vi "S4GUI_003.vi"(7 "Tab ObsEng":enum32{"Obs", "CCD modes", "Guider", "Eng"}(tab)) -> ()   [LabVIEW 2018] (continued)
            n4857 = call-dynamic "Write Interface.vi"("error in (no error)"=w11578, "Interface.lvclass"=w11579, "Channel in"=w11595) -> ("error out"=w11573:errorcluster, "Channel out"=w11572:refnum<class "Channel.lvclass">)  [unwired: 7 in]
            n4858 = call "Write section_name.vi"("error in (no error)"=w11573, "section_name"="CCD_ACS1", "Channel in"=w11572) -> ("error out"=w11574:errorcluster, "Channel out"=w11569:refnum<class "Channel.lvclass">)  [unwired: 7 in]
            n4859 = call-dynamic "save config.vi"("error in (no error)"=w11574, "file config"="lastsaved.cfg", "Channel in"=w11569) -> ("error out"=w11562:errorcluster, "Channel out"=w11563:refnum<class "Channel.lvclass">)  [unwired: 7 in]
            n4860 = call-dynamic "Read State Machine.vi"("error in (no error)"=w11562, "Device in"=w11563) -> ("error out"=w11577:errorcluster, "State Machine.lvclass"=w11567:refnum<class "State Machine.lvclass">, "Device out"=w11568:refnum<class "Channel.lvclass">)  [unwired: 7 in]
            n4861 = call-dynamic "Write State.vi"("error in (no error)"=w11577, "State"=60, "State Machine in"=w11567) -> ("error out"=w11576:errorcluster, "State Machine out"=w11566:refnum<class "State Machine.lvclass">)  [unwired: 7 in]
            n4862 = call-dynamic "Write State Machine.vi"("error in (no error)"=w11576, "State Machine.lvclass"=w11566, "Device in"=w11568) -> ("error out"=w11564:errorcluster, "Device out"=w11565:refnum<class "Channel.lvclass">)  [unwired: 7 in]
            n4863 = call-dynamic "Write Channel.vi"("error in (no error)"=w11564, "Channel.lvclass"=w11565, "Acquisition in"=w11594) -> ("error out"=w11591:errorcluster, "Acquisition out"=w11590:refnum<class "Acquisition.lvclass">)  [unwired: 7 in]
          }
        }
        n4864 = call-dynamic "Write AcquisitionA.vi"("error in (no error)"=w11298, "Acquisition.lvclass"=w11299, "S4ACS_GUI in"=w11281) -> ("error out"=w11285:errorcluster, "S4ACS_GUI out"=w11280:refnum<class "S4GUI.lvclass">)  [unwired: 7 in]
        n4865 = call "Write AcquisitionB.vi"("error in (no error)"=w11296, "Acquisition.lvclass"=w11297, "S4ACS_GUI in"=w11280) -> ("error out"=w11284:errorcluster, "S4ACS_GUI out"=w11279:refnum<class "S4GUI.lvclass">)  [unwired: 7 in]
        n4866 = call-dynamic "Write AcquisitionC.vi"("error in (no error)"=w11294, "Acquisition.lvclass"=w11295, "S4ACS_GUI in"=w11279) -> ("error out"=w11283:errorcluster, "S4ACS_GUI out"=w11278:refnum<class "S4GUI.lvclass">)  [unwired: 7 in]
        n4867 = call-dynamic "Write AcquisitionD.vi"("error in (no error)"=w11286, "Acquisition.lvclass"=w11287, "S4ACS_GUI in"=w11278) -> ("error out"=w11282:errorcluster, "S4ACS_GUI out"=w11262:refnum<class "S4GUI.lvclass">)  [unwired: 7 in]
        n4868 = Merge Errors(w11285, w11284, w11283, w11282) -> (w11261:errorcluster)
        n4869 = call "Read Instrument.lvclass.vi"("error in (no error)"=w11261, "S4ACS_GUI in"=w11262) -> ("error out"=w11267:errorcluster, "Instrument.lvclass"=w11266:refnum<class "Instrument.lvclass">, "S4ACS_GUI out"=w11263:refnum<class "S4GUI.lvclass">)  [unwired: 7 in]
        n4870 = call "Read ASEL.vi"("error in (no error)"=w11267, "Instrument in"=w11266) -> ("error out"=w11274:errorcluster, "Opt_Selector.lvclass"=w11273:refnum<class "Opt_Selector.lvclass">, "Instrument out"=w11272:refnum<class "Instrument.lvclass">)  [unwired: 7 in]
        n4871 = call "Read target name.vi"("error in (no error)"=w11274, "Optics in"=w11273) -> ("error out"=w11270:errorcluster, "target name"=w11250:string, "Optics out"=w11271:refnum<class "Opt_Selector.lvclass">)  [unwired: 7 in]
        n4872 = call "Write ASEL.vi"("error in (no error)"=w11270, "Opt_Selector.lvclass"=w11271, "Instrument in"=w11272) -> ("error out"=w11269:errorcluster, "Instrument out"=w11265:refnum<class "Instrument.lvclass">)  [unwired: 7 in]
        n4873 = Concatenate Strings(w11252, " ASEL=" ("string"), w11250) -> (w11247:string)
        n4874 = case shown="\"ON\"" w11250 {
          tunnel: w11269 -> [w11416 w11427]
          tunnel: [w11416 w11423] -> w11268
          tunnel: w11265 -> [w11415 w11428]
          tunnel: [w11415 w11424] -> w11264
          frame Default {
          }
          frame "ON" {
            n4875 = call "Read WPROT.vi"("error in (no error)"=w11427, "Instrument in"=w11428) -> ("error out"=w11419:errorcluster, "Opt_Selector.lvclass"=w11426:refnum<class "Opt_Selector.lvclass">, "Instrument out"=w11425:refnum<class "Instrument.lvclass">)  [unwired: 7 in]
            n4876 = call-dynamic "Read sequencia.vi"("error in (no error)"=w11419, "Opt_Selector in"=w11426) -> ("error out"=w11418:errorcluster, "sequencia"=w11422:u16, "Opt_Selector out"=w11421:refnum<class "Opt_Selector.lvclass">)  [unwired: 7 in]
            n4877 = case shown="0" w11422 {
              tunnel: w11421 -> [w11430 w11439]
              tunnel: [w11430 w11435] -> w11420
              tunnel: w11418 -> [w11429 w11438]
              tunnel: [w11429 w11433] -> w11417
              frame Default {
              }
              frame 0 {
                n4878 = call-dynamic "Write sequencia.vi"("error in (no error)"=w11438, "sequencia"=u16 1, "Opt_Selector in"=w11439) -> ("error out"=w11434:errorcluster, "Opt_Selector out"=w11436:refnum<class "Opt_Selector.lvclass">)  [unwired: 7 in]
                n4879 = local write "P0"(TRUE ("P0")) -> ()
                n4880 = call-dynamic "Write sequencia_ant.vi"("error in (no error)"=w11434, "sequencia_ant"=u16 1, "Opt_Selector in"=w11436) -> ("error out"=w11433:errorcluster, "Opt_Selector out"=w11435:refnum<class "Opt_Selector.lvclass">)  [unwired: 7 in]
              }
            }
            n4881 = call "Write WPROT.vi"("error in (no error)"=w11417, "Opt_Selector.lvclass"=w11420, "Instrument in"=w11425) -> ("error out"=w11423:errorcluster, "Instrument out"=w11424:refnum<class "Instrument.lvclass">)  [unwired: 7 in]
          }
        }
        n4882 = call "Write Instrument.lvclass.vi"("error in (no error)"=w11268, "Instrument.lvclass"=w11264, "S4ACS_GUI in"=w11263) -> ("error out"=w11248:errorcluster, "S4ACS_GUI out"=w11249:refnum<class "S4GUI.lvclass">)  [unwired: 7 in]
        n4883 = call-dynamic "Write User Event.vi"("error in (no error)"=w11248, "User Event"=w11247, "S4GUI in"=w11249) -> ("error out"=w11245:errorcluster, "S4GUI out"=w11246:refnum<class "S4GUI.lvclass">)  [unwired: 7 in]
      }
      event "Init mode": Value Change {
        n4884 = event-data() -> ()  [unwired: 1 in, 4 out]
        n4885 = call-dynamic "Write User Event.vi"("error in (no error)"=w11648, "User Event"="INIT INSTRUMENT CLICKED", "S4GUI in"=w11649) -> ("error out"=w11646:errorcluster, "S4GUI out"=w11647:refnum<class "S4GUI.lvclass">)  [unwired: 7 in]
        n4886 = call-dynamic "Read Obs_state.vi"("error in (no error)"=w11646, "S4ACS_GUI in"=w11647) -> ("error out"=w11650:errorcluster, "Obs_state"=w11652:u32, "S4ACS_GUI out"=w11653:refnum<class "S4GUI.lvclass">)  [unwired: 7 in]
        n4887 = In Range and Coerce(upper limit=u32 226, x=w11652, lower limit=u32 220 ("upper limit")) -> (In Range?=w11651:bool)  [unwired: 1 out]
        n4888 = case shown="False" w11651 {
          tunnel: [w11661 w11669] -> w11657
          tunnel: [w11660 w11667] -> w11656
          tunnel: w11650 -> [w11659 w11668]
          tunnel: w11653 -> [w11658 w11670]
          frame False {
            n4889 = call-dynamic "Write sync.vi"("error in (no error)"=w11659, "sync"=TRUE, "S4ACS_GUI in"=w11658) -> ("error out"=w11663:errorcluster, "S4ACS_GUI out"=w11662:refnum<class "S4GUI.lvclass">)  [unwired: 7 in]
            n4890 = call-dynamic "Write Obs_state.vi"("error in (no error)"=w11663, "Obs_state"=u32 220, "S4ACS_GUI in"=w11662) -> ("error out"=w11660:errorcluster, "S4ACS_GUI out"=w11661:refnum<class "S4GUI.lvclass">)  [unwired: 7 in]
          }
          frame True {
            n4891 = call-dynamic "Write Obs_state.vi"("error in (no error)"=w11668, "Obs_state"=u32 0, "S4ACS_GUI in"=w11670) -> ("error out"=w11667:errorcluster, "S4ACS_GUI out"=w11669:refnum<class "S4GUI.lvclass">)  [unwired: 7 in]
          }
        }
      }
      event "exit": Value Change {
        n4892 = event-data() -> ()  [unwired: 1 in, 4 out]
        n4893 = call-dynamic "Read Obs_state.vi"("error in (no error)"=w11674, "S4ACS_GUI in"=w11675) -> ("error out"=w11672:errorcluster, "Obs_state"=w11676:u32, "S4ACS_GUI out"=w11673:refnum<class "S4GUI.lvclass">)  [unwired: 7 in]
        n4894 = In Range and Coerce(upper limit=u32 239, x=w11676, lower limit=u32 230 ("upper limit")) -> (In Range?=w11671:bool)  [unwired: 1 out]
        n4895 = case shown="False" w11671 {
          tunnel: [w11689 w11821] -> w11680
          tunnel: [w11688 w11820] -> w11679
          tunnel: w11673 -> [w11682 w11821]
          tunnel: w11672 -> [w11681 w11820]
          frame False {
            n4896 = call "Read Instrument.lvclass.vi"("error in (no error)"=w11681, "S4ACS_GUI in"=w11682) -> ("error out"=w11683:errorcluster, "Instrument.lvclass"=w11685:refnum<class "Instrument.lvclass">, "S4ACS_GUI out"=w11687:refnum<class "S4GUI.lvclass">)  [unwired: 7 in]
            n4897 = call-dynamic "Read operational.vi"("error in (no error)"=w11683, "Server in"=w11685) -> ("error out"=w11686:errorcluster, "operational"=w11684:bool)  [unwired: 7 in, 1 out]
            n4898 = case shown="True" w11684 {
              tunnel: [w11699 w11767] -> w11689
              tunnel: [w11698 w11766] -> w11688
              tunnel: w11687 -> [w11696 w11765]
              tunnel: w11686 -> [w11697 w11764]
              frame False {
                # "Park condition:\nidle: T\nAND\nall discon: F"
                # "S4ICS not operational: only ACS parking can \nbe allowed, depending on its status..."
                n4899 = call-dynamic "VerifyAcqStatus.vi"("error in (no error)"=w11697, "S4GUI in"=w11696) -> ("error out"=w11691:errorcluster, "idle"=w11695:bool, "S4GUI out"=w11693:refnum<class "S4GUI.lvclass">)  [unwired: 6 in, 1 out]
                n4900 = case shown="True" w11695 {
                  selector: w11695 -> [w11700 _]
                  tunnel: [w11700 w11703] -> w11694
                  tunnel: w11693 -> [w11702 w11707]
                  tunnel: [w11702 w11706] -> w11692
                  tunnel: w11691 -> [w11701 w11705]
                  tunnel: [w11701 w11704] -> w11690
                  frame False {
                  }
                  frame True {
                    n4901 = call-dynamic "VerifAllChanDiscon.vi"("error in (no error)"=w11705, "S4GUI in"=w11707) -> ("error out"=w11704:errorcluster, "All disconnected"=w11708:bool, "S4GUI out"=w11706:refnum<class "S4GUI.lvclass">)  [unwired: 7 in]
                    n4902 = Not(x=w11708) -> (.not. x?=w11703:bool)
                  }
                }
                n4903 = case shown="False" w11694 {
                  tunnel: w11690 -> [w11717 w11736]
                  tunnel: w11692 -> [w11718 w11735]
                  tunnel: [w11711 w11734] -> w11699
                  tunnel: [w11710 w11733] -> w11698
                  frame False {
                    # "Acquisition in progress OR no channel operational..."
                    n4904 = Two Button Dialog(message="Parking not possible.\nAre you sure to quit?", 2:"Yes" ("T button name (\"OK\")")) -> (T button?=w11714:bool)  [unwired: 1 in]
                    n4905 = case shown="True" w11714 {
                      tunnel: [w11721 w11725] -> w11713
                      tunnel: w11718 -> [w11721 w11726]
                      tunnel: w11717 -> [w11720 w11724]
                      tunnel: [w11720 w11723] -> w11712
                      tunnel: ["EXIT CLICKED WITH NO PARKING POSSIBLE. EXIT CANCELLED. " ("T button name (\"OK\")") "EXIT CLICKED WITH NO PARKING POSSIBLE." ("T button name (\"OK\")")] -> w11709
                      frame False {
                        # "NO (cancel)"
                      }
                      frame True {
                        # "YES"
                        n4906 = call-dynamic "Write exit.vi"("error in (no error)"=w11724, "exit"=TRUE, "S4GUI in"=w11726) -> ("error out"=w11723:errorcluster, "S4GUI out"=w11725:refnum<class "S4GUI.lvclass">)  [unwired: 7 in]
                      }
                    }
                    n4907 = call-dynamic "Write User Event.vi"("error in (no error)"=w11712, "User Event"=w11709, "S4GUI in"=w11713) -> ("error out"=w11710:errorcluster, "S4GUI out"=w11711:refnum<class "S4GUI.lvclass">)  [unwired: 7 in]
                  }
                  frame True {
                    # "No acquisition in progress."
                    n4908 = call <vilib>:"Three Button Dialog.vi"("Right Button Text (\"Cancel\")"="Cancel" ("Right Button Text (\"Cancel\")"), "Center Button Text (\"No\")"="NO" ("F button name (\"Cancel\")"), "Left Button Text (\"Yes\")"="YES" ("T button name (\"OK\")"), "message"="Instrument parking not possible.\nPark acquisition system before exiting?") -> ("Which Button?"=w11731:T34)  [unwired: 7 in]
                    n4909 = case shown="\"Right Button\", Default" w11731 {
                      tunnel: w11736 -> [w11743 w11747 w11756]
                      tunnel: w11735 -> [w11742 w11748 w11755]
                      tunnel: [w11739 w11746 w11752] -> w11734
                      tunnel: [w11737 w11745 w11750] -> w11733
                      frame "Center Button" {
                        # "NO"
                        n4910 = call-dynamic "Write exit.vi"("error in (no error)"=w11743, "exit"=TRUE, "S4GUI in"=w11742) -> ("error out"=w11738:errorcluster, "S4GUI out"=w11740:refnum<class "S4GUI.lvclass">)  [unwired: 7 in]
                        n4911 = call-dynamic "Write User Event.vi"("error in (no error)"=w11738, "User Event"="EXIT APP CLICKED WITH NO PARKING.", "S4GUI in"=w11740) -> ("error out"=w11737:errorcluster, "S4GUI out"=w11739:refnum<class "S4GUI.lvclass">)  [unwired: 7 in]
                      }
                      frame "Right Button", Default {
                        # "CANCEL"
                        n4912 = call-dynamic "Write User Event.vi"("error in (no error)"=w11747, "User Event"="EXIT APP CLICKED, BUT CANCELLED BY USER.", "S4GUI in"=w11748) -> ("error out"=w11745:errorcluster, "S4GUI out"=w11746:refnum<class "S4GUI.lvclass">)  [unwired: 7 in]
                      }
                      frame "Left Button" {
                        # "YES"
                        n4913 = call-dynamic "Write sync.vi"("error in (no error)"=w11756, "sync"=TRUE, "S4ACS_GUI in"=w11755) -> ("error out"=w11758:errorcluster, "S4ACS_GUI out"=w11757:refnum<class "S4GUI.lvclass">)  [unwired: 7 in]
                        n4914 = call-dynamic "Write Obs_state.vi"("error in (no error)"=w11758, "Obs_state"=u32 232, "S4ACS_GUI in"=w11757) -> ("error out"=w11751:errorcluster, "S4ACS_GUI out"=w11753:refnum<class "S4GUI.lvclass">)  [unwired: 7 in]
                        n4915 = call-dynamic "Write User Event.vi"("error in (no error)"=w11751, "User Event"="EXIT APP CLICKED AND ONLY ACS PARKING PROCEDURE DONE.", "S4GUI in"=w11753) -> ("error out"=w11750:errorcluster, "S4GUI out"=w11752:refnum<class "S4GUI.lvclass">)  [unwired: 7 in]
                      }
                    }
                  }
                }
              }
              frame True {
                # "Park condition:\nidle: T"
                # "S4ICS operational: Instrument parking allowed \nand verifying ACS channels status..."
                n4916 = call-dynamic "VerifyAcqStatus.vi"("error in (no error)"=w11764, "S4GUI in"=w11765) -> ("error out"=w11761:errorcluster, "idle"=w11762:bool, "S4GUI out"=w11763:refnum<class "S4GUI.lvclass">)  [unwired: 6 in, 1 out]
                n4917 = case shown="False" w11762 {
                  tunnel: [w11771 w11795] -> w11767
                  tunnel: [w11770 w11794] -> w11766
                  tunnel: w11763 -> [w11769 w11788]
                  tunnel: w11761 -> [w11768 w11787]
                  frame False {
                    # "Acquisition in progress..."
                    n4918 = Two Button Dialog(message="Parking not possible.\nAre you sure to quit?", 2:"Yes" ("T button name (\"OK\")")) -> (T button?=w11775:bool)  [unwired: 1 in]
                    n4919 = case shown="True" w11775 {
                      tunnel: [w11780 w11784] -> w11774
                      tunnel: w11769 -> [w11780 w11785]
                      tunnel: w11768 -> [w11779 w11783]
                      tunnel: [w11779 w11782] -> w11773
                      tunnel: ["EXIT CLICKED WITH NO PARKING POSSIBLE. EXIT CANCELLED. " ("T button name (\"OK\")") "EXIT CLICKED WITH NO PARKING POSSIBLE." ("T button name (\"OK\")")] -> w11772
                      frame False {
                        # "NO (cancel)"
                      }
                      frame True {
                        # "YES"
                        n4920 = call-dynamic "Write exit.vi"("error in (no error)"=w11783, "exit"=TRUE, "S4GUI in"=w11785) -> ("error out"=w11782:errorcluster, "S4GUI out"=w11784:refnum<class "S4GUI.lvclass">)  [unwired: 7 in]
                      }
                    }
                    n4921 = call-dynamic "Write User Event.vi"("error in (no error)"=w11773, "User Event"=w11772, "S4GUI in"=w11774) -> ("error out"=w11770:errorcluster, "S4GUI out"=w11771:refnum<class "S4GUI.lvclass">)  [unwired: 7 in]
                  }
                  frame True {
                    # "Acquisition system in IDLE state."
                    n4922 = call <vilib>:"Three Button Dialog.vi"("Right Button Text (\"Cancel\")"="Cancel" ("Right Button Text (\"Cancel\")"), "Center Button Text (\"No\")"="NO" ("F button name (\"Cancel\")"), "Left Button Text (\"Yes\")"="YES" ("T button name (\"OK\")"), "message"="Park before exiting?") -> ("Which Button?"=w11790:T34)  [unwired: 7 in]
                    n4923 = case shown="\"Left Button\"" w11790 {
                      tunnel: w11787 -> [w11802 w11806 w11816]
                      tunnel: w11788 -> [w11801 w11807 w11815]
                      tunnel: [w11798 w11805 w11812] -> w11795
                      tunnel: [w11796 w11804 w11810] -> w11794
                      frame "Center Button" {
                        # "NO"
                        n4924 = call-dynamic "Write exit.vi"("error in (no error)"=w11802, "exit"=TRUE, "S4GUI in"=w11801) -> ("error out"=w11797:errorcluster, "S4GUI out"=w11799:refnum<class "S4GUI.lvclass">)  [unwired: 7 in]
                        n4925 = call-dynamic "Write User Event.vi"("error in (no error)"=w11797, "User Event"="EXIT APP CLICKED WITH NO PARKING.", "S4GUI in"=w11799) -> ("error out"=w11796:errorcluster, "S4GUI out"=w11798:refnum<class "S4GUI.lvclass">)  [unwired: 7 in]
                      }
                      frame "Right Button", Default {
                        # "CANCEL"
                        n4926 = call-dynamic "Write User Event.vi"("error in (no error)"=w11806, "User Event"="EXIT APP CLICKED, BUT CANCELLED BY USER.", "S4GUI in"=w11807) -> ("error out"=w11804:errorcluster, "S4GUI out"=w11805:refnum<class "S4GUI.lvclass">)  [unwired: 7 in]
                      }
                      frame "Left Button" {
                        # "YES"
                        n4927 = call-dynamic "Write sync.vi"("error in (no error)"=w11816, "sync"=TRUE, "S4ACS_GUI in"=w11815) -> ("error out"=w11818:errorcluster, "S4ACS_GUI out"=w11817:refnum<class "S4GUI.lvclass">)  [unwired: 7 in]
                        n4928 = call-dynamic "Write Obs_state.vi"("error in (no error)"=w11818, "Obs_state"=u32 230, "S4ACS_GUI in"=w11817) -> ("error out"=w11811:errorcluster, "S4ACS_GUI out"=w11813:refnum<class "S4GUI.lvclass">)  [unwired: 7 in]
                        n4929 = call-dynamic "Write User Event.vi"("error in (no error)"=w11811, "User Event"="EXIT APP CLICKED AND PARKING PROCEDURE DONE.", "S4GUI in"=w11813) -> ("error out"=w11810:errorcluster, "S4GUI out"=w11812:refnum<class "S4GUI.lvclass">)  [unwired: 7 in]
                      }
                    }
                  }
                }
              }
            }
          }
          frame True {
            # "Parking already in progress..."
          }
        }
      }
      event "WPSEL_stop": Value Change {
        n4930 = event-data() -> ()  [unwired: 1 in, 4 out]
        n4931 = call "Read Instrument.lvclass.vi"("error in (no error)"=w11840, "S4ACS_GUI in"=w11841) -> ("error out"=w11838:errorcluster, "Instrument.lvclass"=w11839:refnum<class "Instrument.lvclass">, "S4ACS_GUI out"=w11825:refnum<class "S4GUI.lvclass">)  [unwired: 7 in]
        n4932 = call "Read WPSEL.vi"("error in (no error)"=w11838, "Instrument in"=w11839) -> ("error out"=w11834:errorcluster, "Opt_Selector.lvclass"=w11837:refnum<class "Opt_Selector.lvclass">, "Instrument out"=w11828:refnum<class "Instrument.lvclass">)  [unwired: 7 in]
        n4933 = call-dynamic "Read State Machine.vi"("error in (no error)"=w11834, "Device in"=w11837) -> ("error out"=w11833:errorcluster, "State Machine.lvclass"=w11836:refnum<class "State Machine.lvclass">, "Device out"=w11830:refnum<class "Opt_Selector.lvclass">)  [unwired: 7 in]
        n4934 = call "Next State.vi"("error in (no error)"=w11833, "New_State"=10, "State Machine in"=w11836) -> ("error out"=w11832:errorcluster, "State Machine out"=w11831:refnum<class "State Machine.lvclass">)  [unwired: 7 in]
        n4935 = call-dynamic "Write State Machine.vi"("error in (no error)"=w11832, "State Machine.lvclass"=w11831, "Device in"=w11830) -> ("error out"=w11827:errorcluster, "Device out"=w11829:refnum<class "Opt_Selector.lvclass">)  [unwired: 7 in]
        n4936 = call "Write WPSEL.vi"("error in (no error)"=w11827, "Opt_Selector.lvclass"=w11829, "Instrument in"=w11828) -> ("error out"=w11824:errorcluster, "Instrument out"=w11826:refnum<class "Instrument.lvclass">)  [unwired: 7 in]
        n4937 = call "Write Instrument.lvclass.vi"("error in (no error)"=w11824, "Instrument.lvclass"=w11826, "S4ACS_GUI in"=w11825) -> ("error out"=w11823:errorcluster, "S4ACS_GUI out"=w11822:refnum<class "S4GUI.lvclass">)  [unwired: 7 in]
      }
      event "WPSEL_init": Value Change {
        n4938 = event-data() -> ()  [unwired: 1 in, 4 out]
        n4939 = call "Read Instrument.lvclass.vi"("error in (no error)"=w11860, "S4ACS_GUI in"=w11861) -> ("error out"=w11858:errorcluster, "Instrument.lvclass"=w11859:refnum<class "Instrument.lvclass">, "S4ACS_GUI out"=w11845:refnum<class "S4GUI.lvclass">)  [unwired: 7 in]
        n4940 = call "Read WPSEL.vi"("error in (no error)"=w11858, "Instrument in"=w11859) -> ("error out"=w11854:errorcluster, "Opt_Selector.lvclass"=w11857:refnum<class "Opt_Selector.lvclass">, "Instrument out"=w11848:refnum<class "Instrument.lvclass">)  [unwired: 7 in]
        n4941 = call-dynamic "Read State Machine.vi"("error in (no error)"=w11854, "Device in"=w11857) -> ("error out"=w11853:errorcluster, "State Machine.lvclass"=w11856:refnum<class "State Machine.lvclass">, "Device out"=w11850:refnum<class "Opt_Selector.lvclass">)  [unwired: 7 in]
        n4942 = call "Next State.vi"("error in (no error)"=w11853, "New_State"=30, "State Machine in"=w11856) -> ("error out"=w11852:errorcluster, "State Machine out"=w11851:refnum<class "State Machine.lvclass">)  [unwired: 7 in]
        n4943 = call-dynamic "Write State Machine.vi"("error in (no error)"=w11852, "State Machine.lvclass"=w11851, "Device in"=w11850) -> ("error out"=w11847:errorcluster, "Device out"=w11849:refnum<class "Opt_Selector.lvclass">)  [unwired: 7 in]
        n4944 = call "Write WPSEL.vi"("error in (no error)"=w11847, "Opt_Selector.lvclass"=w11849, "Instrument in"=w11848) -> ("error out"=w11844:errorcluster, "Instrument out"=w11846:refnum<class "Instrument.lvclass">)  [unwired: 7 in]
        n4945 = call "Write Instrument.lvclass.vi"("error in (no error)"=w11844, "Instrument.lvclass"=w11846, "S4ACS_GUI in"=w11845) -> ("error out"=w11843:errorcluster, "S4ACS_GUI out"=w11842:refnum<class "S4GUI.lvclass">)  [unwired: 7 in]
      }
      event "GMIR_target": Value Change {
        n4946 = event-data() -> ("NewVal"=w11871:dbl)  [unwired: 1 in, 3 out]
        n4947 = call "Read Instrument.lvclass.vi"("error in (no error)"=w11875, "S4ACS_GUI in"=w11876) -> ("error out"=w11873:errorcluster, "Instrument.lvclass"=w11874:refnum<class "Instrument.lvclass">, "S4ACS_GUI out"=w11865:refnum<class "S4GUI.lvclass">)  [unwired: 7 in]
        n4948 = call "Read GMIR.vi"("error in (no error)"=w11873, "Instrument in"=w11874) -> ("error out"=w11870:errorcluster, "Opt_Continuous.lvclass"=w11872:refnum<class "Opt_Continuous.lvclass">, "Instrument out"=w11868:refnum<class "Instrument.lvclass">)  [unwired: 7 in]
        n4949 = call "Write target.vi"("error in (no error)"=w11870, "target"=w11871, "Optics in"=w11872) -> ("error out"=w11867:errorcluster, "Optics out"=w11869:refnum<class "Opt_Continuous.lvclass">)  [unwired: 7 in]
        n4950 = call "Write GMIR.vi"("error in (no error)"=w11867, "Opt_Continuous.lvclass"=w11869, "Instrument in"=w11868) -> ("error out"=w11864:errorcluster, "Instrument out"=w11866:refnum<class "Instrument.lvclass">)  [unwired: 7 in]
        n4951 = call "Write Instrument.lvclass.vi"("error in (no error)"=w11864, "Instrument.lvclass"=w11866, "S4ACS_GUI in"=w11865) -> ("error out"=w11863:errorcluster, "S4ACS_GUI out"=w11862:refnum<class "S4GUI.lvclass">)  [unwired: 7 in]
      }
      event "GMIR_target 2": Value Change {
        n4952 = event-data() -> ("NewVal"=w11878:dbl)  [unwired: 1 in, 3 out]
        n4953 = call-dynamic "Read GSserver.lvclass.vi"("error in (no error)"=w11891, "S4GUI in"=w11892) -> ("error out"=w11889:errorcluster, "GSserver.lvclass"=w11890:refnum<class "GSserver.lvclass">, "S4GUI out"=w11886:refnum<class "S4GUI.lvclass">)  [unwired: 7 in]
        n4954 = call-dynamic "Read Mirror.vi"("error in (no error)"=w11889, "GSserver in"=w11890) -> ("error out"=w11880:errorcluster, "GSdevice.lvclass"=w11882:refnum<class "GSdevice.lvclass">, "GSserver out"=w11888:refnum<class "GSserver.lvclass">)  [unwired: 7 in]
        n4955 = Number To Fractional String(number=w11878) -> (F-format string=w11877:string)  [unwired: 3 in]
        n4956 = call-dynamic "Write target.vi"("error in (no error)"=w11880, "target"=w11877, "GSdevice in"=w11882) -> ("error out"=w11879:errorcluster, "GSdevice out"=w11881:refnum<class "GSdevice.lvclass">)  [unwired: 7 in]
        n4957 = call-dynamic "Write Mirror.vi"("error in (no error)"=w11879, "GSdevice.lvclass"=w11881, "GSserver in"=w11888) -> ("error out"=w11885:errorcluster, "GSserver out"=w11887:refnum<class "GSserver.lvclass">)  [unwired: 7 in]
        n4958 = call-dynamic "Write GSserver.lvclass.vi"("error in (no error)"=w11885, "GSserver.lvclass"=w11887, "S4GUI in"=w11886) -> ("error out"=w11884:errorcluster, "S4GUI out"=w11883:refnum<class "S4GUI.lvclass">)  [unwired: 7 in]
      }
      event "GMIR_set": Value Change {
        n4959 = event-data() -> ()  [unwired: 1 in, 4 out]
        n4960 = call "Read Instrument.lvclass.vi"("error in (no error)"=w11911, "S4ACS_GUI in"=w11912) -> ("error out"=w11909:errorcluster, "Instrument.lvclass"=w11910:refnum<class "Instrument.lvclass">, "S4ACS_GUI out"=w11898:refnum<class "S4GUI.lvclass">)  [unwired: 7 in]
        n4961 = call "Read GMIR.vi"("error in (no error)"=w11909, "Instrument in"=w11910) -> ("error out"=w11906:errorcluster, "Opt_Continuous.lvclass"=w11908:refnum<class "Opt_Continuous.lvclass">, "Instrument out"=w11900:refnum<class "Instrument.lvclass">)  [unwired: 7 in]
        n4962 = call-dynamic "Read State Machine.vi"("error in (no error)"=w11906, "Device in"=w11908) -> ("error out"=w11905:errorcluster, "State Machine.lvclass"=w11896:refnum<class "State Machine.lvclass">, "Device out"=w11902:refnum<class "Opt_Continuous.lvclass">)  [unwired: 7 in]
        n4963 = call "Next State.vi"("error in (no error)"=w11905, "New_State"=1, "State Machine in"=w11896) -> ("error out"=w11904:errorcluster, "State Machine out"=w11903:refnum<class "State Machine.lvclass">)  [unwired: 7 in]
        n4964 = call-dynamic "Write State Machine.vi"("error in (no error)"=w11904, "State Machine.lvclass"=w11903, "Device in"=w11902) -> ("error out"=w11899:errorcluster, "Device out"=w11901:refnum<class "Opt_Continuous.lvclass">)  [unwired: 7 in]
        n4965 = call "Write GMIR.vi"("error in (no error)"=w11899, "Opt_Continuous.lvclass"=w11901, "Instrument in"=w11900) -> ("error out"=w11893:errorcluster, "Instrument out"=w11894:refnum<class "Instrument.lvclass">)  [unwired: 7 in]
        n4966 = call "Write Instrument.lvclass.vi"("error in (no error)"=w11893, "Instrument.lvclass"=w11894, "S4ACS_GUI in"=w11898) -> ("error out"=w11897:errorcluster, "S4ACS_GUI out"=w11895:refnum<class "S4GUI.lvclass">)  [unwired: 7 in]
      }
      event "GMIR_set 2": Value Change {
        n4967 = event-data() -> ()  [unwired: 1 in, 4 out]
        n4968 = call-dynamic "Read GSserver.lvclass.vi"("error in (no error)"=w11931, "S4GUI in"=w11932) -> ("error out"=w11929:errorcluster, "GSserver.lvclass"=w11930:refnum<class "GSserver.lvclass">, "S4GUI out"=w11918:refnum<class "S4GUI.lvclass">)  [unwired: 7 in]
        n4969 = call-dynamic "Read Mirror.vi"("error in (no error)"=w11929, "GSserver in"=w11930) -> ("error out"=w11926:errorcluster, "GSdevice.lvclass"=w11928:refnum<class "GSdevice.lvclass">, "GSserver out"=w11920:refnum<class "GSserver.lvclass">)  [unwired: 7 in]
        n4970 = call-dynamic "Read State Machine.vi"("error in (no error)"=w11926, "Device in"=w11928) -> ("error out"=w11925:errorcluster, "State Machine.lvclass"=w11916:refnum<class "State Machine.lvclass">, "Device out"=w11922:refnum<class "GSdevice.lvclass">)  [unwired: 7 in]
        n4971 = call "Next State.vi"("error in (no error)"=w11925, "New_State"=10, "State Machine in"=w11916) -> ("error out"=w11924:errorcluster, "State Machine out"=w11923:refnum<class "State Machine.lvclass">)  [unwired: 7 in]
        n4972 = call-dynamic "Write State Machine.vi"("error in (no error)"=w11924, "State Machine.lvclass"=w11923, "Device in"=w11922) -> ("error out"=w11919:errorcluster, "Device out"=w11921:refnum<class "GSdevice.lvclass">)  [unwired: 7 in]
        n4973 = call-dynamic "Write Mirror.vi"("error in (no error)"=w11919, "GSdevice.lvclass"=w11921, "GSserver in"=w11920) -> ("error out"=w11913:errorcluster, "GSserver out"=w11914:refnum<class "GSserver.lvclass">)  [unwired: 7 in]
        n4974 = call-dynamic "Write GSserver.lvclass.vi"("error in (no error)"=w11913, "GSserver.lvclass"=w11914, "S4GUI in"=w11918) -> ("error out"=w11917:errorcluster, "S4GUI out"=w11915:refnum<class "S4GUI.lvclass">)  [unwired: 7 in]
      }
      event "GMIR_stop", "GMIR_stop 2": Value Change {
        n4975 = event-data() -> ()  [unwired: 1 in, 4 out]
        n4976 = call "Read Instrument.lvclass.vi"("error in (no error)"=w11951, "S4ACS_GUI in"=w11952) -> ("error out"=w11949:errorcluster, "Instrument.lvclass"=w11950:refnum<class "Instrument.lvclass">, "S4ACS_GUI out"=w11936:refnum<class "S4GUI.lvclass">)  [unwired: 7 in]
        n4977 = call "Read GMIR.vi"("error in (no error)"=w11949, "Instrument in"=w11950) -> ("error out"=w11945:errorcluster, "Opt_Continuous.lvclass"=w11948:refnum<class "Opt_Continuous.lvclass">, "Instrument out"=w11939:refnum<class "Instrument.lvclass">)  [unwired: 7 in]
        n4978 = call-dynamic "Read State Machine.vi"("error in (no error)"=w11945, "Device in"=w11948) -> ("error out"=w11944:errorcluster, "State Machine.lvclass"=w11947:refnum<class "State Machine.lvclass">, "Device out"=w11941:refnum<class "Opt_Continuous.lvclass">)  [unwired: 7 in]
        n4979 = call "Next State.vi"("error in (no error)"=w11944, "New_State"=10, "State Machine in"=w11947) -> ("error out"=w11943:errorcluster, "State Machine out"=w11942:refnum<class "State Machine.lvclass">)  [unwired: 7 in]
        n4980 = call-dynamic "Write State Machine.vi"("error in (no error)"=w11943, "State Machine.lvclass"=w11942, "Device in"=w11941) -> ("error out"=w11938:errorcluster, "Device out"=w11940:refnum<class "Opt_Continuous.lvclass">)  [unwired: 7 in]
        n4981 = call "Write GMIR.vi"("error in (no error)"=w11938, "Opt_Continuous.lvclass"=w11940, "Instrument in"=w11939) -> ("error out"=w11935:errorcluster, "Instrument out"=w11937:refnum<class "Instrument.lvclass">)  [unwired: 7 in]
        n4982 = call "Write Instrument.lvclass.vi"("error in (no error)"=w11935, "Instrument.lvclass"=w11937, "S4ACS_GUI in"=w11936) -> ("error out"=w11934:errorcluster, "S4ACS_GUI out"=w11933:refnum<class "S4GUI.lvclass">)  [unwired: 7 in]
      }
      event "GMIR_init": Value Change {
        n4983 = event-data() -> ()  [unwired: 1 in, 4 out]
        n4984 = call "Read Instrument.lvclass.vi"("error in (no error)"=w11971, "S4ACS_GUI in"=w11972) -> ("error out"=w11969:errorcluster, "Instrument.lvclass"=w11970:refnum<class "Instrument.lvclass">, "S4ACS_GUI out"=w11956:refnum<class "S4GUI.lvclass">)  [unwired: 7 in]
        n4985 = call "Read GMIR.vi"("error in (no error)"=w11969, "Instrument in"=w11970) -> ("error out"=w11965:errorcluster, "Opt_Continuous.lvclass"=w11968:refnum<class "Opt_Continuous.lvclass">, "Instrument out"=w11959:refnum<class "Instrument.lvclass">)  [unwired: 7 in]
        n4986 = call-dynamic "Read State Machine.vi"("error in (no error)"=w11965, "Device in"=w11968) -> ("error out"=w11964:errorcluster, "State Machine.lvclass"=w11967:refnum<class "State Machine.lvclass">, "Device out"=w11961:refnum<class "Opt_Continuous.lvclass">)  [unwired: 7 in]
        n4987 = call "Next State.vi"("error in (no error)"=w11964, "New_State"=30, "State Machine in"=w11967) -> ("error out"=w11963:errorcluster, "State Machine out"=w11962:refnum<class "State Machine.lvclass">)  [unwired: 7 in]
        n4988 = call-dynamic "Write State Machine.vi"("error in (no error)"=w11963, "State Machine.lvclass"=w11962, "Device in"=w11961) -> ("error out"=w11958:errorcluster, "Device out"=w11960:refnum<class "Opt_Continuous.lvclass">)  [unwired: 7 in]
        n4989 = call "Write GMIR.vi"("error in (no error)"=w11958, "Opt_Continuous.lvclass"=w11960, "Instrument in"=w11959) -> ("error out"=w11955:errorcluster, "Instrument out"=w11957:refnum<class "Instrument.lvclass">)  [unwired: 7 in]
        n4990 = call "Write Instrument.lvclass.vi"("error in (no error)"=w11955, "Instrument.lvclass"=w11957, "S4ACS_GUI in"=w11956) -> ("error out"=w11954:errorcluster, "S4ACS_GUI out"=w11953:refnum<class "S4GUI.lvclass">)  [unwired: 7 in]
      }
      event "GFOC_target": Value Change {
        n4991 = event-data() -> ("NewVal"=w11982:dbl)  [unwired: 1 in, 3 out]
        n4992 = call "Read Instrument.lvclass.vi"("error in (no error)"=w11986, "S4ACS_GUI in"=w11987) -> ("error out"=w11984:errorcluster, "Instrument.lvclass"=w11985:refnum<class "Instrument.lvclass">, "S4ACS_GUI out"=w11976:refnum<class "S4GUI.lvclass">)  [unwired: 7 in]
        n4993 = call "Read GFOC.vi"("error in (no error)"=w11984, "Instrument in"=w11985) -> ("error out"=w11981:errorcluster, "Opt_Continuous.lvclass"=w11983:refnum<class "Opt_Continuous.lvclass">, "Instrument out"=w11979:refnum<class "Instrument.lvclass">)  [unwired: 7 in]
        n4994 = call "Write target.vi"("error in (no error)"=w11981, "target"=w11982, "Optics in"=w11983) -> ("error out"=w11978:errorcluster, "Optics out"=w11980:refnum<class "Opt_Continuous.lvclass">)  [unwired: 7 in]
        n4995 = call "Write GFOC.vi"("error in (no error)"=w11978, "Opt_Continuous.lvclass"=w11980, "Instrument in"=w11979) -> ("error out"=w11975:errorcluster, "Instrument out"=w11977:refnum<class "Instrument.lvclass">)  [unwired: 7 in]
        n4996 = call "Write Instrument.lvclass.vi"("error in (no error)"=w11975, "Instrument.lvclass"=w11977, "S4ACS_GUI in"=w11976) -> ("error out"=w11974:errorcluster, "S4ACS_GUI out"=w11973:refnum<class "S4GUI.lvclass">)  [unwired: 7 in]
      }
      event "GFOC_target 2": Value Change {
        n4997 = event-data() -> ("NewVal"=w11989:dbl)  [unwired: 1 in, 3 out]
        n4998 = call-dynamic "Read GSserver.lvclass.vi"("error in (no error)"=w12002, "S4GUI in"=w12003) -> ("error out"=w12000:errorcluster, "GSserver.lvclass"=w12001:refnum<class "GSserver.lvclass">, "S4GUI out"=w11993:refnum<class "S4GUI.lvclass">)  [unwired: 7 in]
        n4999 = call-dynamic "Read Focus.vi"("error in (no error)"=w12000, "GSserver in"=w12001) -> ("error out"=w11998:errorcluster, "GSdevice.lvclass"=w11999:refnum<class "GSdevice.lvclass">, "GSserver out"=w11996:refnum<class "GSserver.lvclass">)  [unwired: 7 in]
        n5000 = Number To Fractional String(number=w11989) -> (F-format string=w11988:string)  [unwired: 3 in]
        n5001 = call-dynamic "Write target.vi"("error in (no error)"=w11998, "target"=w11988, "GSdevice in"=w11999) -> ("error out"=w11995:errorcluster, "GSdevice out"=w11997:refnum<class "GSdevice.lvclass">)  [unwired: 7 in]
        n5002 = call-dynamic "Write Focus.vi"("error in (no error)"=w11995, "GSdevice.lvclass"=w11997, "GSserver in"=w11996) -> ("error out"=w11992:errorcluster, "GSserver out"=w11994:refnum<class "GSserver.lvclass">)  [unwired: 7 in]
        n5003 = call-dynamic "Write GSserver.lvclass.vi"("error in (no error)"=w11992, "GSserver.lvclass"=w11994, "S4GUI in"=w11993) -> ("error out"=w11991:errorcluster, "S4GUI out"=w11990:refnum<class "S4GUI.lvclass">)  [unwired: 7 in]
      }
      event "GFOC_set": Value Change {
        n5004 = event-data() -> ()  [unwired: 1 in, 4 out]
        n5005 = call "Read Instrument.lvclass.vi"("error in (no error)"=w12022, "S4ACS_GUI in"=w12023) -> ("error out"=w12020:errorcluster, "Instrument.lvclass"=w12021:refnum<class "Instrument.lvclass">, "S4ACS_GUI out"=w12008:refnum<class "S4GUI.lvclass">)  [unwired: 7 in]
        n5006 = call "Read GFOC.vi"("error in (no error)"=w12020, "Instrument in"=w12021) -> ("error out"=w12017:errorcluster, "Opt_Continuous.lvclass"=w12019:refnum<class "Opt_Continuous.lvclass">, "Instrument out"=w12011:refnum<class "Instrument.lvclass">)  [unwired: 7 in]
        n5007 = call-dynamic "Read State Machine.vi"("error in (no error)"=w12017, "Device in"=w12019) -> ("error out"=w12016:errorcluster, "State Machine.lvclass"=w12005:refnum<class "State Machine.lvclass">, "Device out"=w12013:refnum<class "Opt_Continuous.lvclass">)  [unwired: 7 in]
        n5008 = call "Next State.vi"("error in (no error)"=w12016, "New_State"=1, "State Machine in"=w12005) -> ("error out"=w12015:errorcluster, "State Machine out"=w12014:refnum<class "State Machine.lvclass">)  [unwired: 7 in]
        n5009 = call-dynamic "Write State Machine.vi"("error in (no error)"=w12015, "State Machine.lvclass"=w12014, "Device in"=w12013) -> ("error out"=w12010:errorcluster, "Device out"=w12012:refnum<class "Opt_Continuous.lvclass">)  [unwired: 7 in]
        n5010 = call "Write GFOC.vi"("error in (no error)"=w12010, "Opt_Continuous.lvclass"=w12012, "Instrument in"=w12011) -> ("error out"=w12007:errorcluster, "Instrument out"=w12009:refnum<class "Instrument.lvclass">)  [unwired: 7 in]
        n5011 = call "Write Instrument.lvclass.vi"("error in (no error)"=w12007, "Instrument.lvclass"=w12009, "S4ACS_GUI in"=w12008) -> ("error out"=w12006:errorcluster, "S4ACS_GUI out"=w12004:refnum<class "S4GUI.lvclass">)  [unwired: 7 in]
      }
      event "GFOC_set 2": Value Change {
        n5012 = event-data() -> ()  [unwired: 1 in, 4 out]
        n5013 = call-dynamic "Read GSserver.lvclass.vi"("error in (no error)"=w12042, "S4GUI in"=w12043) -> ("error out"=w12040:errorcluster, "GSserver.lvclass"=w12041:refnum<class "GSserver.lvclass">, "S4GUI out"=w12028:refnum<class "S4GUI.lvclass">)  [unwired: 7 in]
        n5014 = call-dynamic "Read Focus.vi"("error in (no error)"=w12040, "GSserver in"=w12041) -> ("error out"=w12037:errorcluster, "GSdevice.lvclass"=w12039:refnum<class "GSdevice.lvclass">, "GSserver out"=w12031:refnum<class "GSserver.lvclass">)  [unwired: 7 in]
        n5015 = call-dynamic "Read State Machine.vi"("error in (no error)"=w12037, "Device in"=w12039) -> ("error out"=w12036:errorcluster, "State Machine.lvclass"=w12025:refnum<class "State Machine.lvclass">, "Device out"=w12033:refnum<class "GSdevice.lvclass">)  [unwired: 7 in]
        n5016 = call "Next State.vi"("error in (no error)"=w12036, "New_State"=10, "State Machine in"=w12025) -> ("error out"=w12035:errorcluster, "State Machine out"=w12034:refnum<class "State Machine.lvclass">)  [unwired: 7 in]
        n5017 = call-dynamic "Write State Machine.vi"("error in (no error)"=w12035, "State Machine.lvclass"=w12034, "Device in"=w12033) -> ("error out"=w12030:errorcluster, "Device out"=w12032:refnum<class "GSdevice.lvclass">)  [unwired: 7 in]
        n5018 = call-dynamic "Write Focus.vi"("error in (no error)"=w12030, "GSdevice.lvclass"=w12032, "GSserver in"=w12031) -> ("error out"=w12027:errorcluster, "GSserver out"=w12029:refnum<class "GSserver.lvclass">)  [unwired: 7 in]
        n5019 = call-dynamic "Write GSserver.lvclass.vi"("error in (no error)"=w12027, "GSserver.lvclass"=w12029, "S4GUI in"=w12028) -> ("error out"=w12026:errorcluster, "S4GUI out"=w12024:refnum<class "S4GUI.lvclass">)  [unwired: 7 in]
      }
      event "GFOC_stop", "GFOC_stop 2": Value Change {
        n5020 = event-data() -> ()  [unwired: 1 in, 4 out]
        n5021 = call "Read Instrument.lvclass.vi"("error in (no error)"=w12062, "S4ACS_GUI in"=w12063) -> ("error out"=w12060:errorcluster, "Instrument.lvclass"=w12061:refnum<class "Instrument.lvclass">, "S4ACS_GUI out"=w12047:refnum<class "S4GUI.lvclass">)  [unwired: 7 in]
        n5022 = call "Read GFOC.vi"("error in (no error)"=w12060, "Instrument in"=w12061) -> ("error out"=w12056:errorcluster, "Opt_Continuous.lvclass"=w12059:refnum<class "Opt_Continuous.lvclass">, "Instrument out"=w12050:refnum<class "Instrument.lvclass">)  [unwired: 7 in]
        n5023 = call-dynamic "Read State Machine.vi"("error in (no error)"=w12056, "Device in"=w12059) -> ("error out"=w12055:errorcluster, "State Machine.lvclass"=w12058:refnum<class "State Machine.lvclass">, "Device out"=w12052:refnum<class "Opt_Continuous.lvclass">)  [unwired: 7 in]
        n5024 = call "Next State.vi"("error in (no error)"=w12055, "New_State"=10, "State Machine in"=w12058) -> ("error out"=w12054:errorcluster, "State Machine out"=w12053:refnum<class "State Machine.lvclass">)  [unwired: 7 in]
        n5025 = call-dynamic "Write State Machine.vi"("error in (no error)"=w12054, "State Machine.lvclass"=w12053, "Device in"=w12052) -> ("error out"=w12049:errorcluster, "Device out"=w12051:refnum<class "Opt_Continuous.lvclass">)  [unwired: 7 in]
        n5026 = call "Write GFOC.vi"("error in (no error)"=w12049, "Opt_Continuous.lvclass"=w12051, "Instrument in"=w12050) -> ("error out"=w12046:errorcluster, "Instrument out"=w12048:refnum<class "Instrument.lvclass">)  [unwired: 7 in]
        n5027 = call "Write Instrument.lvclass.vi"("error in (no error)"=w12046, "Instrument.lvclass"=w12048, "S4ACS_GUI in"=w12047) -> ("error out"=w12045:errorcluster, "S4ACS_GUI out"=w12044:refnum<class "S4GUI.lvclass">)  [unwired: 7 in]
      }
      event "GFOC_init": Value Change {
        n5028 = event-data() -> ()  [unwired: 1 in, 4 out]
        n5029 = call "Read Instrument.lvclass.vi"("error in (no error)"=w12082, "S4ACS_GUI in"=w12083) -> ("error out"=w12080:errorcluster, "Instrument.lvclass"=w12081:refnum<class "Instrument.lvclass">, "S4ACS_GUI out"=w12067:refnum<class "S4GUI.lvclass">)  [unwired: 7 in]
        n5030 = call "Read GFOC.vi"("error in (no error)"=w12080, "Instrument in"=w12081) -> ("error out"=w12076:errorcluster, "Opt_Continuous.lvclass"=w12079:refnum<class "Opt_Continuous.lvclass">, "Instrument out"=w12070:refnum<class "Instrument.lvclass">)  [unwired: 7 in]
        n5031 = call-dynamic "Read State Machine.vi"("error in (no error)"=w12076, "Device in"=w12079) -> ("error out"=w12075:errorcluster, "State Machine.lvclass"=w12078:refnum<class "State Machine.lvclass">, "Device out"=w12072:refnum<class "Opt_Continuous.lvclass">)  [unwired: 7 in]
        n5032 = call "Next State.vi"("error in (no error)"=w12075, "New_State"=30, "State Machine in"=w12078) -> ("error out"=w12074:errorcluster, "State Machine out"=w12073:refnum<class "State Machine.lvclass">)  [unwired: 7 in]
        n5033 = call-dynamic "Write State Machine.vi"("error in (no error)"=w12074, "State Machine.lvclass"=w12073, "Device in"=w12072) -> ("error out"=w12069:errorcluster, "Device out"=w12071:refnum<class "Opt_Continuous.lvclass">)  [unwired: 7 in]
        n5034 = call "Write GFOC.vi"("error in (no error)"=w12069, "Opt_Continuous.lvclass"=w12071, "Instrument in"=w12070) -> ("error out"=w12066:errorcluster, "Instrument out"=w12068:refnum<class "Instrument.lvclass">)  [unwired: 7 in]
        n5035 = call "Write Instrument.lvclass.vi"("error in (no error)"=w12066, "Instrument.lvclass"=w12068, "S4ACS_GUI in"=w12067) -> ("error out"=w12065:errorcluster, "S4ACS_GUI out"=w12064:refnum<class "S4GUI.lvclass">)  [unwired: 7 in]
      }
      event "CALW_target": Value Change {
        n5036 = event-data() -> ("NewVal"=w12093:dbl)  [unwired: 1 in, 3 out]
        n5037 = call "Read Instrument.lvclass.vi"("error in (no error)"=w12097, "S4ACS_GUI in"=w12098) -> ("error out"=w12095:errorcluster, "Instrument.lvclass"=w12096:refnum<class "Instrument.lvclass">, "S4ACS_GUI out"=w12087:refnum<class "S4GUI.lvclass">)  [unwired: 7 in]
        n5038 = call "Read CALW.vi"("error in (no error)"=w12095, "Instrument in"=w12096) -> ("error out"=w12092:errorcluster, "Opt_Selector.lvclass"=w12094:refnum<class "Opt_Selector.lvclass">, "Instrument out"=w12090:refnum<class "Instrument.lvclass">)  [unwired: 7 in]
        n5039 = call "Write target.vi"("error in (no error)"=w12092, "target"=w12093, "Optics in"=w12094) -> ("error out"=w12089:errorcluster, "Optics out"=w12091:refnum<class "Opt_Selector.lvclass">)  [unwired: 7 in]
        n5040 = call "Write CALW.vi"("error in (no error)"=w12089, "Opt_Selector.lvclass"=w12091, "Instrument in"=w12090) -> ("error out"=w12086:errorcluster, "Instrument out"=w12088:refnum<class "Instrument.lvclass">)  [unwired: 7 in]
        n5041 = call "Write Instrument.lvclass.vi"("error in (no error)"=w12086, "Instrument.lvclass"=w12088, "S4ACS_GUI in"=w12087) -> ("error out"=w12085:errorcluster, "S4ACS_GUI out"=w12084:refnum<class "S4GUI.lvclass">)  [unwired: 7 in]
      }
      event "CALW_set": Value Change {
        n5042 = event-data() -> ()  [unwired: 1 in, 4 out]
        n5043 = call "Read Instrument.lvclass.vi"("error in (no error)"=w12117, "S4ACS_GUI in"=w12118) -> ("error out"=w12115:errorcluster, "Instrument.lvclass"=w12116:refnum<class "Instrument.lvclass">, "S4ACS_GUI out"=w12103:refnum<class "S4GUI.lvclass">)  [unwired: 7 in]
        n5044 = call "Read CALW.vi"("error in (no error)"=w12115, "Instrument in"=w12116) -> ("error out"=w12112:errorcluster, "Opt_Selector.lvclass"=w12114:refnum<class "Opt_Selector.lvclass">, "Instrument out"=w12106:refnum<class "Instrument.lvclass">)  [unwired: 7 in]
        n5045 = call-dynamic "Read State Machine.vi"("error in (no error)"=w12112, "Device in"=w12114) -> ("error out"=w12111:errorcluster, "State Machine.lvclass"=w12100:refnum<class "State Machine.lvclass">, "Device out"=w12108:refnum<class "Opt_Selector.lvclass">)  [unwired: 7 in]
        n5046 = call "Next State.vi"("error in (no error)"=w12111, "New_State"=1, "State Machine in"=w12100) -> ("error out"=w12110:errorcluster, "State Machine out"=w12109:refnum<class "State Machine.lvclass">)  [unwired: 7 in]
        n5047 = call-dynamic "Write State Machine.vi"("error in (no error)"=w12110, "State Machine.lvclass"=w12109, "Device in"=w12108) -> ("error out"=w12105:errorcluster, "Device out"=w12107:refnum<class "Opt_Selector.lvclass">)  [unwired: 7 in]
        n5048 = call "Write CALW.vi"("error in (no error)"=w12105, "Opt_Selector.lvclass"=w12107, "Instrument in"=w12106) -> ("error out"=w12102:errorcluster, "Instrument out"=w12104:refnum<class "Instrument.lvclass">)  [unwired: 7 in]
        n5049 = call "Write Instrument.lvclass.vi"("error in (no error)"=w12102, "Instrument.lvclass"=w12104, "S4ACS_GUI in"=w12103) -> ("error out"=w12101:errorcluster, "S4ACS_GUI out"=w12099:refnum<class "S4GUI.lvclass">)  [unwired: 7 in]
      }
      event "CALW_stop": Value Change {
        n5050 = event-data() -> ()  [unwired: 1 in, 4 out]
        n5051 = call "Read Instrument.lvclass.vi"("error in (no error)"=w12137, "S4ACS_GUI in"=w12138) -> ("error out"=w12135:errorcluster, "Instrument.lvclass"=w12136:refnum<class "Instrument.lvclass">, "S4ACS_GUI out"=w12122:refnum<class "S4GUI.lvclass">)  [unwired: 7 in]
        n5052 = call "Read CALW.vi"("error in (no error)"=w12135, "Instrument in"=w12136) -> ("error out"=w12131:errorcluster, "Opt_Selector.lvclass"=w12134:refnum<class "Opt_Selector.lvclass">, "Instrument out"=w12125:refnum<class "Instrument.lvclass">)  [unwired: 7 in]
        n5053 = call-dynamic "Read State Machine.vi"("error in (no error)"=w12131, "Device in"=w12134) -> ("error out"=w12130:errorcluster, "State Machine.lvclass"=w12133:refnum<class "State Machine.lvclass">, "Device out"=w12127:refnum<class "Opt_Selector.lvclass">)  [unwired: 7 in]
        n5054 = call "Next State.vi"("error in (no error)"=w12130, "New_State"=10, "State Machine in"=w12133) -> ("error out"=w12129:errorcluster, "State Machine out"=w12128:refnum<class "State Machine.lvclass">)  [unwired: 7 in]
        n5055 = call-dynamic "Write State Machine.vi"("error in (no error)"=w12129, "State Machine.lvclass"=w12128, "Device in"=w12127) -> ("error out"=w12124:errorcluster, "Device out"=w12126:refnum<class "Opt_Selector.lvclass">)  [unwired: 7 in]
        n5056 = call "Write CALW.vi"("error in (no error)"=w12124, "Opt_Selector.lvclass"=w12126, "Instrument in"=w12125) -> ("error out"=w12121:errorcluster, "Instrument out"=w12123:refnum<class "Instrument.lvclass">)  [unwired: 7 in]
        n5057 = call "Write Instrument.lvclass.vi"("error in (no error)"=w12121, "Instrument.lvclass"=w12123, "S4ACS_GUI in"=w12122) -> ("error out"=w12120:errorcluster, "S4ACS_GUI out"=w12119:refnum<class "S4GUI.lvclass">)  [unwired: 7 in]
      }
      event "CALW_init": Value Change {
        n5058 = event-data() -> ()  [unwired: 1 in, 4 out]
        n5059 = call "Read Instrument.lvclass.vi"("error in (no error)"=w12157, "S4ACS_GUI in"=w12158) -> ("error out"=w12155:errorcluster, "Instrument.lvclass"=w12156:refnum<class "Instrument.lvclass">, "S4ACS_GUI out"=w12142:refnum<class "S4GUI.lvclass">)  [unwired: 7 in]
        n5060 = call "Read CALW.vi"("error in (no error)"=w12155, "Instrument in"=w12156) -> ("error out"=w12151:errorcluster, "Opt_Selector.lvclass"=w12154:refnum<class "Opt_Selector.lvclass">, "Instrument out"=w12145:refnum<class "Instrument.lvclass">)  [unwired: 7 in]
        n5061 = call-dynamic "Read State Machine.vi"("error in (no error)"=w12151, "Device in"=w12154) -> ("error out"=w12150:errorcluster, "State Machine.lvclass"=w12153:refnum<class "State Machine.lvclass">, "Device out"=w12147:refnum<class "Opt_Selector.lvclass">)  [unwired: 7 in]
        n5062 = call "Next State.vi"("error in (no error)"=w12150, "New_State"=30, "State Machine in"=w12153) -> ("error out"=w12149:errorcluster, "State Machine out"=w12148:refnum<class "State Machine.lvclass">)  [unwired: 7 in]
        n5063 = call-dynamic "Write State Machine.vi"("error in (no error)"=w12149, "State Machine.lvclass"=w12148, "Device in"=w12147) -> ("error out"=w12144:errorcluster, "Device out"=w12146:refnum<class "Opt_Selector.lvclass">)  [unwired: 7 in]
        n5064 = call "Write CALW.vi"("error in (no error)"=w12144, "Opt_Selector.lvclass"=w12146, "Instrument in"=w12145) -> ("error out"=w12141:errorcluster, "Instrument out"=w12143:refnum<class "Instrument.lvclass">)  [unwired: 7 in]
        n5065 = call "Write Instrument.lvclass.vi"("error in (no error)"=w12141, "Instrument.lvclass"=w12143, "S4ACS_GUI in"=w12142) -> ("error out"=w12140:errorcluster, "S4ACS_GUI out"=w12139:refnum<class "S4GUI.lvclass">)  [unwired: 7 in]
      }
      event "ASEL_target": Value Change {
        n5066 = event-data() -> ("NewVal"=w12168:dbl)  [unwired: 1 in, 3 out]
        n5067 = call "Read Instrument.lvclass.vi"("error in (no error)"=w12172, "S4ACS_GUI in"=w12173) -> ("error out"=w12170:errorcluster, "Instrument.lvclass"=w12171:refnum<class "Instrument.lvclass">, "S4ACS_GUI out"=w12162:refnum<class "S4GUI.lvclass">)  [unwired: 7 in]
